vi "GDSAPI_CloneMethod.vi"(8 "error in (no error)":errorcluster, 9 "DestinationClassPath(*.lvclass)":path, 10 "SourceClassMethod(*.vi)":path, 11 "SourceClassPath(*.lvclass)":path) -> (0 "error out":errorcluster, 3 "CreatedMethodPathOut":path)   [LabVIEW 2014]
doc: "This VI creates Methods in a class."
uses:
  <resource>/Framework/Providers/Open_GDS/ClassProviders/Provider_LvNativeClass/ClassWriterNative_class/ClassWriterNative.lvclass
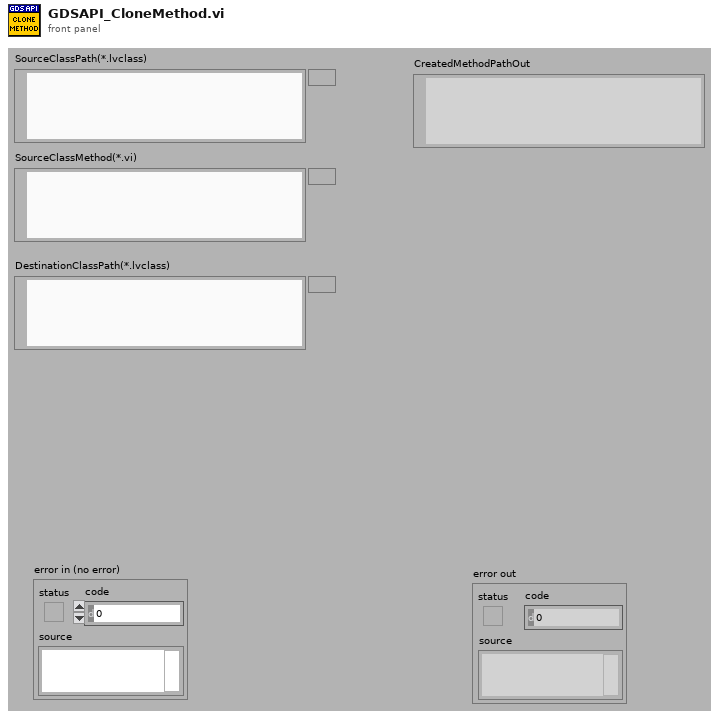
[diagram p1: front panel]
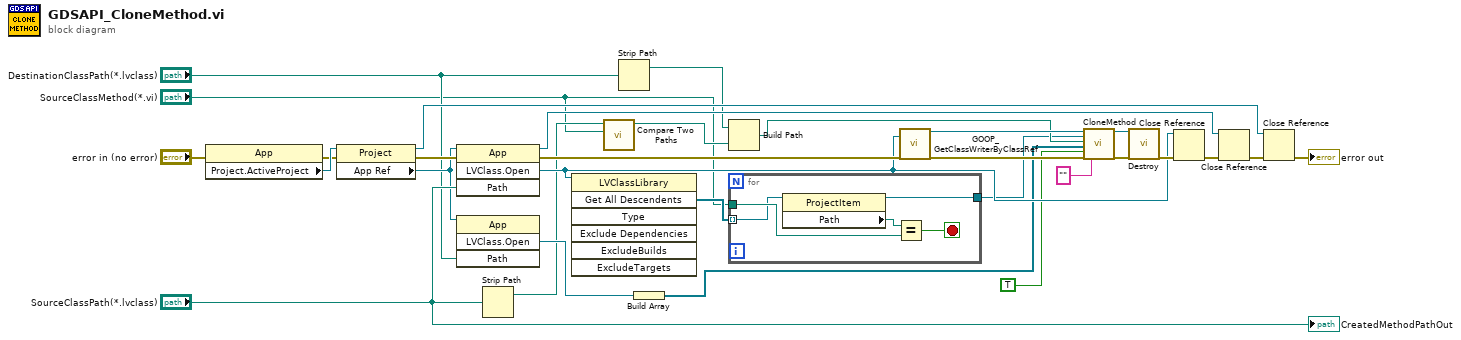
[diagram p0: block diagram]
diagram:
  n1 = property class="App"(error in="error in (no error)") -> (error out=w27:errorcluster, "Project.ActiveProject"=w28:refnum<vi>)  [unwired: 1 in, 1 out]
  n2 = property class="Project"(reference=w28, error in=w27) -> (reference out=w22:refnum<vi>, error out=w15:errorcluster, "App Ref"=w9:refnum<vi>)
  n3 = invoke class="App" method="LVClass.Open"(reference=w9, error in=w15, "Path"="SourceClassPath(*.lvclass)") -> (reference out=w24:refnum<vi>, error out=w29:errorcluster, "LVClass.Open"=w13:refnum<vi>)  [unwired: 1 in, 1 out]
  n4 = invoke class="App" method="LVClass.Open"(reference=w9, "Path"="DestinationClassPath(*.lvclass)") -> ("LVClass.Open"=w7:refnum<vi>)  [unwired: 2 in, 3 out]
  n5 = Strip Path(path="SourceClassPath(*.lvclass)") -> (stripped path=w2:path)  [unwired: 1 out]
  n6 = invoke class="LVClassLibrary" method="Get All Descendents"(reference=w13) -> ("All Descendents"=w14:refnum<vi>[])  [unwired: 6 in, 6 out]
  n7 = call <vilib>:"Compare Two Paths.vi"("Path 2"="SourceClassMethod(*.vi)", "Path 1"=w2) -> ("Relative Path from 1 to 2"=w11:path)  [unwired: 6 in, 3 out]
  n8 = Strip Path(path="DestinationClassPath(*.lvclass)") -> (stripped path=w12:path)  [unwired: 1 out]
  n9 = Build Array(w7) -> (w6:refnum<vi>[])
  n10 = Build Path(base path=w12, name or relative path=w11) -> (appended path=w10:path)
  n11 = for {
    tunnel: w14 -> [w31] mode=indexing
    tunnel: "SourceClassMethod(*.vi)" -> [w34]
    tunnel: [w32] -> w4
    stop <- w33 stop-if-true
    n12 = property class="ProjectItem"(reference=w31) -> (reference out=w32:refnum<vi>, "Path"=w35:path)  [unwired: 1 in, 1 out]
    n13 = Equal?(x=w35, y=w34) -> (x = y?=w33:bool)
  }
  n14 = call <resource>:"GOOP_GetClassWriterByClassRef.vi"("LVClassLibrary Refnum"=w13, "error in (no error)"=w29) -> ("ClassWriterNative.lvclass"=w18:refnum<class "ClassWriterNative.lvclass">, "error out"=w20:errorcluster)  [unwired: 16 in]
  n15 = call-dynamic "CloneMethod.vi"("ClassWriterNative.lvclass"=w18, "VIItemRefIn"=w4, "NewVIPath"=w10, "LibraryOwners"=w6, "OpenVIWhenDone"=TRUE, "error in (no error)"=w20, "ViDescription"="") -> ("ClassWriterNative.lvclass"=w17:refnum<class "ClassWriterNative.lvclass">, "error out"=w19:errorcluster)  [unwired: 11 in]
  n16 = call-dynamic "Destroy.vi"("ClassWriterNative"=w17, "error in (no error)"=w19) -> ("error out"=w30:errorcluster)  [unwired: 17 in]
  n17 = Close Reference(reference=w13, error in (no error)=w30) -> (error out=w25:errorcluster)
  n18 = Close Reference(reference=w24, error in (no error)=w25) -> (error out=w23:errorcluster)
  n19 = Close Reference(reference=w22, error in (no error)=w23) -> (error out=→"error out":errorcluster)
  "CreatedMethodPathOut" <- "SourceClassPath(*.lvclass)"
